vi "Create.vi"(8 "error in (no error)":errorcluster) -> (0 "error out":errorcluster, 3 "Inherited Tests Filter":refnum<class "Inherited Tests Filter.lvclass">)   [LabVIEW 2020, in "Inherited Tests Filter.lvclass"]
uses:
  Inherited Tests Filter.lvclass
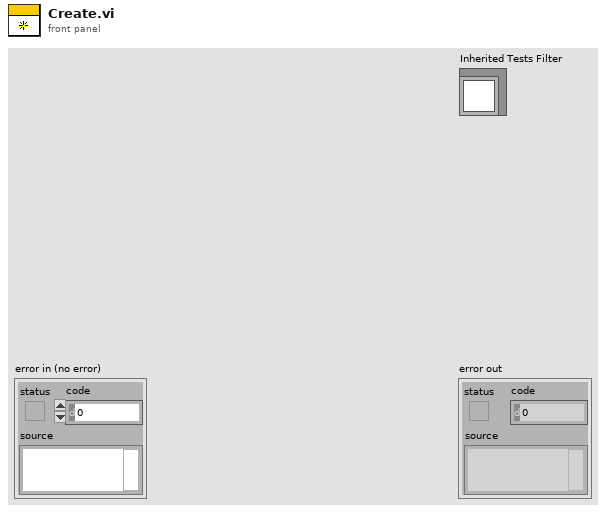
[diagram p1: front panel]
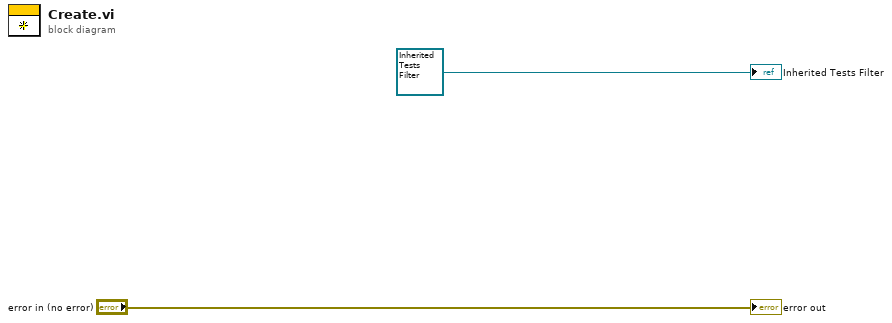
[diagram p0: block diagram]
diagram:
  "error out" <- "error in (no error)"
  "Inherited Tests Filter" <- refnum<class "Inherited Tests Filter.lvclass"> refnum ("Inherited Tests Filter")
